vi "Test Case Indent Correct When Added.vi"(8 "error in (no error)":errorcluster, 11 "Result Model Tests in":refnum<class "Result Model Test Enumeration.lvclass">) -> (0 "error out":errorcluster, 3 "Result Model Tests out":refnum<class "Result Model Test Enumeration.lvclass">)   [LabVIEW 2020, in "Result Model Test Enumeration.lvclass"]
uses:
  Result Model Test Enumeration.lvclass
  C:/Program Files (x86)/National Instruments/LabVIEW 2020/vi.lib/Astemes/LUnit/Test Case.lvclass
  <vilib>/Astemes/LUnit/Test Case.lvclass/Test Case.ctl
  206db1ee-aa99-40b9-8881-171f2a77c34b.vi
  <vilib>/Astemes/LUnit/Palette/Pass.vi
  <vilib>/Astemes/LUnit/Palette/Fail.vi
  <vilib>/Astemes/LUnit/Compare Variants.vi
  <vilib>/Astemes/LUnit/Describe Comparison.vi
  <vilib>/Astemes/LUnit/Set Assertion Type.vi
  <vilib>/Astemes/LUnit/Add test result.vi
  <vilib>/Astemes/LUnit/Variant to string.vi
  <vilib>/Astemes/LUnit/LUnit Record Assertion Result.vi
  <vilib>/Astemes/LUnit/LUnit Aggregate Assertion Results.vi
  <vilib>/Astemes/LUnit/Method Result/LUnit Merge Status.vi
  <vilib>/Astemes/LUnit/LUnit Concatenate result strings.vi
  <vilib>/Utility/Data Type/Get Type Information.vi
  <vilib>/Utility/LVClass/Get LV Class Name.vi
  Framework/Result Model/Result Model.lvclass
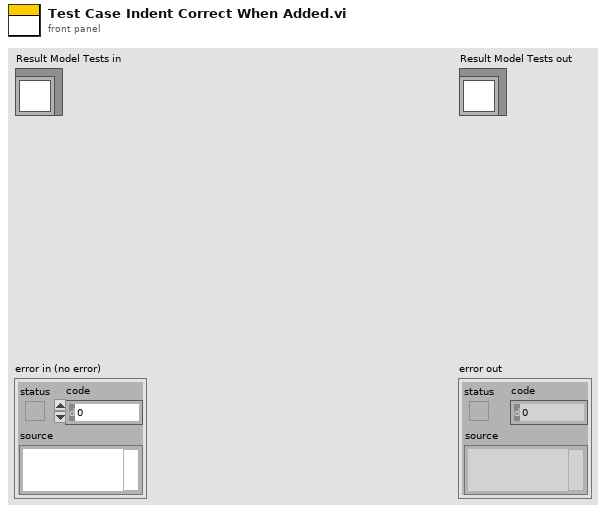
[diagram p1: front panel]
types:
  T1 = cluster{"Left Cell String":string, "Child Text":string[], "Child Tag":string, "Item Indent":i32, "Child Only?":bool, "Glyph Index":i32}[]
  T2 = cluster{"Left Cell String":string, "Child Text":string[], "Child Tag":string, "Item Indent":i32, "Child Only?":bool, "Glyph Index":i32}
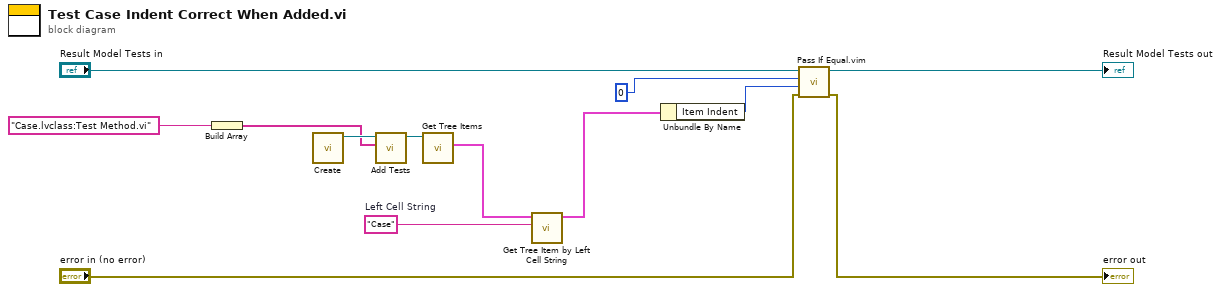
[diagram p0: block diagram]
diagram:
  w3 = "Case"  # Left Cell String
  n1 = Build Array("Case.lvclass:Test Method.vi" ("String")) -> (w6:string[])
  n2 = call "Create.vi"() -> ("Result Model out"=w12:refnum<class "Result Model.lvclass">)  [unwired: 11 in]
  n3 = call "Add Tests.vi"("Tests"=w6, "Result Model In"=w12) -> ("Result Model Out"=w11:refnum<class "Result Model.lvclass">)  [unwired: 9 in]
  n4 = call "Get Tree Items.vi"("Result Model In"=w11) -> ("Tree Items"=w10:T1)  [unwired: 10 in]
  n5 = call "Get Tree Item by Left Cell String.vi"("Left Cell String"=w3, "Tree Items"=w10) -> ("Item"=w8:T2)  [unwired: 9 in]
  n6 = Unbundle By Name(w8) -> ("Item Indent"=w7:i32)
  n7 = call "Pass If Equal.vim"("error in (no error)"="error in (no error)", "Actual"=w7, "Expected"=0 ("Item Indent"), "LUnit Test Case In"="Result Model Tests in") -> ("error out"=→"error out":errorcluster, "LUnit Test Case Out"=→"Result Model Tests out":refnum<class "Result Model Test Enumeration.lvclass">)  [unwired: 6 in]
